vi "Ini key write (Boolean).vi"(7 "Section":string, 8 "error in (no error)":errorcluster, 9 "Values (Boolean)":bool[](array[boolean]), 10 "Ini file interface":T2, 11 "Ini file refnum in":T1) -> (0 "error out":errorcluster, 3 "Ini file refnum out":T1)   [LabVIEW 2020]
uses:
  <vilib>/Utility/config.llb/Config Data RefNum.ctl
  Typedefs/Ini file interface (Boolean).ctl
  <vilib>/Utility/config.llb/Read Key (Boolean).vi
  <vilib>/Utility/config.llb/Write Key (Boolean).vi
  <vilib>/Utility/config.llb/NI_LVConfig.lvlib
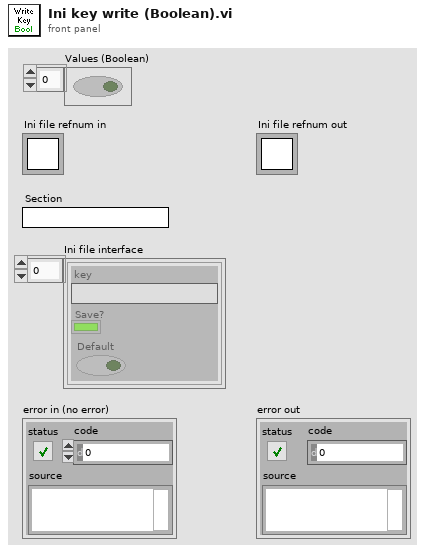
[diagram p1: front panel]
types:
  T1 = typedef "NI_LVConfig.lvlib/Config Data RefNum.ctl" = refnum<k1>
  T2 = typedef "Ini file interface (Boolean).ctl" = cluster{"key":string, "Save?":bool, "Default":bool}[]
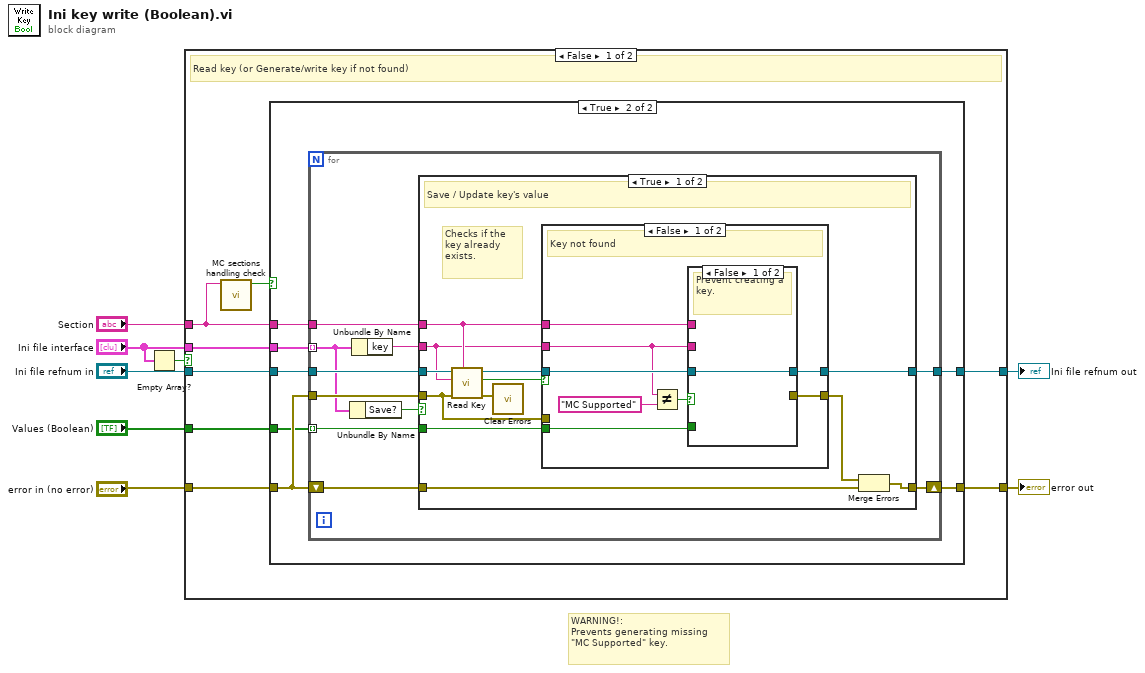
[diagram p0: block diagram]
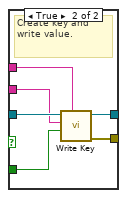
[diagram p3: hidden frame]
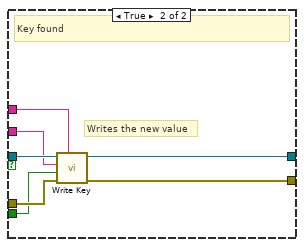
[diagram p4: hidden frame]
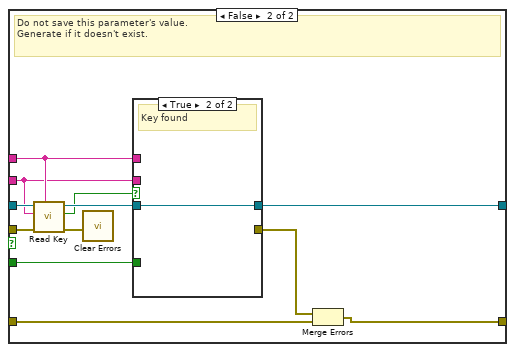
[diagram p5: hidden frame]
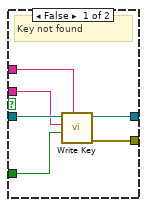
[diagram p6: hidden frame]
diagram:
  # "WARNING!:\nPrevents generating missing \"MC Supported\" key."
  n1 = Empty Array?(array="Ini file interface") -> (empty?=w3:bool)
  n2 = case shown="False" w3 {
    tunnel: "Ini file refnum in" -> [w16 w90]
    tunnel: [w15 w90] -> w8
    tunnel: [w14 w89] -> w7
    tunnel: "error in (no error)" -> [w13 w89]
    tunnel: "Section" -> [w10 _]
    tunnel: "Ini file interface" -> [w12 _]
    tunnel: "Values (Boolean)" -> [w11 _]
    frame False {
      # "Read key (or Generate/write key if not found)"
      n3 = call "MC sections handling check.vi"("Section name"=w10) -> ("Section is \"Initial MovCor Values\" AND MC is supported"=w9:bool)  [unwired: 10 in]
      n4 = case shown="True" w9 {
        tunnel: w16 -> [w18 w25]
        tunnel: [w18 w24] -> w15
        tunnel: [w17 w23] -> w14
        tunnel: w13 -> [w17 w22]
        tunnel: w10 -> [_ w21]
        tunnel: w12 -> [_ w20]
        tunnel: w11 -> [_ w19]
        frame False {
          # "The [Initial MovCor Values] section not handled when the MC UI is unavailable"
        }
        frame True {
          n5 = for {
            tunnel: w25 -> [w35]
            tunnel: w22 -> [w34]
            tunnel: [w33] -> w24
            shift-right: [w32] -> w23
            shift-left: w22 -> [w31]
            tunnel: w20 -> [w27] mode=indexing
            tunnel: w19 -> [w30] mode=indexing
            tunnel: w21 -> [w29]
            n6 = Unbundle By Name(w27) -> ("Save?"=w26:bool)
            n7 = Unbundle By Name(w27) -> ("key"=w28:string)
            n8 = case shown="True" w26 {
              tunnel: w35 -> [w47 w81]
              tunnel: w34 -> [w36 w80]
              tunnel: [w38 w71] -> w33
              tunnel: [w46 w79] -> w32
              tunnel: w31 -> [w45 w78]
              tunnel: w28 -> [w41 w74]
              tunnel: w30 -> [w39 w72]
              tunnel: w29 -> [w42 w75]
              frame True {
                # "Checks if the key already exists."
                # "Save / Update key's value"
                n9 = call-poly <vilib>:"Read Key.vi"("section"=w42, "error in (no error)"=w36, "key"=w41, "refnum"=w47) -> ("error out"=w44:errorcluster, "found?"=w37:bool, "refnum out"=w43:T1)  [unwired: 4 in, 1 out]
                n10 = call <vilib>:"Clear Errors.vi"("error in (no error)"=w44) -> ()  [unwired: 5 in, 2 out]
                n11 = case shown="False" w37 {
                  tunnel: w43 -> [w55 w69]
                  tunnel: [w54 w68] -> w38
                  tunnel: [w53 w66] -> w40
                  tunnel: w42 -> [w52 w65]
                  tunnel: w41 -> [w49 w64]
                  tunnel: w39 -> [w51 w63]
                  tunnel: w36 -> [_ w67]
                  frame False {
                    # "Key not found"
                    n12 = Not Equal?(x=w49, y="MC Supported") -> (x != y?=w48:bool)
                    n13 = case shown="False" w48 {
                      tunnel: w55 -> [w56 w62]
                      tunnel: [w56 w61] -> w54
                      tunnel: [_ w60] -> w53
                      tunnel: w52 -> [_ w59]
                      tunnel: w49 -> [_ w58]
                      tunnel: w51 -> [_ w57]
                      frame False {
                        # "Prevent creating a key."
                      }
                      frame True {
                        # "Create key and write value."
                        n14 = call-poly <vilib>:"Write Key.vi"("section"=w59, "value"=w57, "key"=w58, "refnum"=w62) -> ("error out"=w60:errorcluster, "refnum out"=w61:T1)  [unwired: 5 in, 1 out]
                      }
                    }
                  }
                  frame True {
                    # "Writes the new value"
                    # "Key found"
                    n15 = call-poly <vilib>:"Write Key.vi"("section"=w65, "error in (no error)"=w67, "value"=w63, "key"=w64, "refnum"=w69) -> ("error out"=w66:errorcluster, "refnum out"=w68:T1)  [unwired: 4 in, 1 out]
                  }
                }
                n16 = Merge Errors(w40, w45) -> (w46:errorcluster)
              }
              frame False {
                # "Do not save this parameter's value.\nGenerate if it doesn't exist."
                n17 = call-poly <vilib>:"Read Key.vi"("section"=w75, "error in (no error)"=w80, "key"=w74, "refnum"=w81) -> ("error out"=w77:errorcluster, "found?"=w70:bool, "refnum out"=w76:T1)  [unwired: 4 in, 1 out]
                n18 = call <vilib>:"Clear Errors.vi"("error in (no error)"=w77) -> ()  [unwired: 5 in, 2 out]
                n19 = case shown="True" w70 {
                  tunnel: w76 -> [w87 w88]
                  tunnel: [w86 w88] -> w71
                  tunnel: [w85 _] -> w73
                  tunnel: w75 -> [w84 _]
                  tunnel: w74 -> [w83 _]
                  tunnel: w72 -> [w82 _]
                  frame False {
                    # "Key not found"
                    n20 = call-poly <vilib>:"Write Key.vi"("section"=w84, "value"=w82, "key"=w83, "refnum"=w87) -> ("error out"=w85:errorcluster, "refnum out"=w86:T1)  [unwired: 5 in, 1 out]
                  }
                  frame True {
                    # "Key found"
                  }
                }
                n21 = Merge Errors(w73, w78) -> (w79:errorcluster)
              }
            }
          }
        }
      }
    }
    frame True {
      # "Setup array is empty"
    }
  }
  "Ini file refnum out" <- w8
  "error out" <- w7
